vi "Get GPU Device Information.vi"(8 "error in":errorcluster, 9 "Reset Device?":bool, 10 "Test Device Execution?":bool, 11 "Device ID":T2) -> (0 "error out":errorcluster, 1 "CUDA Driver Version":string, 2 "CUDA Runtime API Version":string, 3 "Device Name":string, 4 "Supports Double Precision?":bool, 5 "Device Properties":T3[](array[typedef]), 7 "Available Devices":i32)   [LabVIEW 2020]
doc: "Investigates GPU devices installed in the system and optionally executes code on one of those devices."
uses:
  <vilib>/addons/lvgpu/lvcuda/CUDA Device (CUdevice).ctl
  <vilib>/addons/lvgpu/lvcuda/CUDA Device Properties (cudaDeviceProp).ctl
  <vilib>/addons/lvgpu/lvcuda.lvlib
  Get GPU Device Information.lvlib
panel:
  out "Status:":string
  in  "UI":T1(tab)
  out "Device Execution Profile":dbl[](graph)
  out "CUDA Build Version":string
  out "Error Help":string
  # "."
  # "The CUDA Runtime API version is the same as the CUDA Toolkit version. When multiple CUDA Toolkit versions are installed on the system, the inputs to Initialize Device or Initialize Library function determine which version is used. \n\nNOTE: This example uses the version selected when running Initialize Device with default inputs."
  # "The CUDA Driver version is determined by the NVIDIA display driver active in the OS."
  # "The CUDA Build version is the version of the CUDA Toolkit on which this toolkit's interface and settings are based."
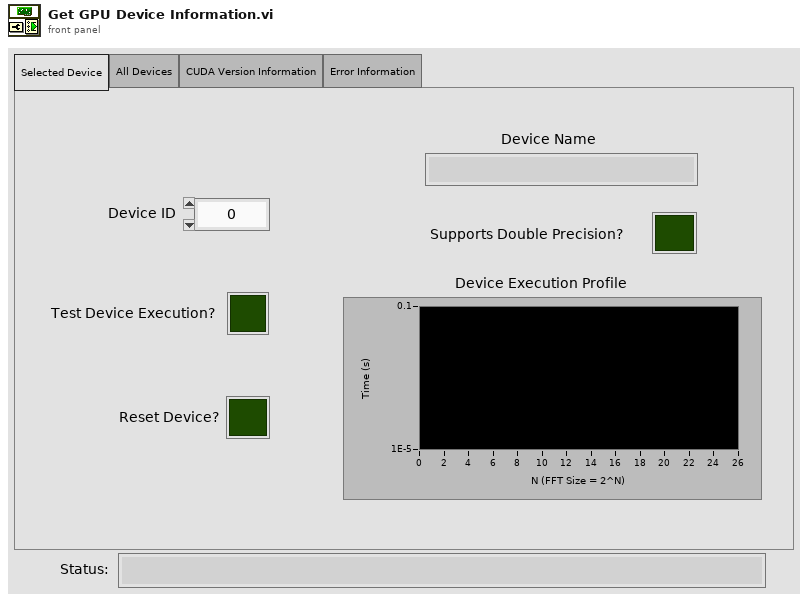
[diagram p1: front panel]
types:
  T1 = enum32{"Selected Device", "All Devices", "CUDA Version Information", "Error Information"}
  T2 = typedef "lvcuda.lvlib/CUDA Device (CUdevice).ctl" = i32
  T3 = typedef "lvcuda.lvlib/CUDA Device Properties (cudaDeviceProp).ctl" = cluster{"Name":string, "Total Global Memory (Bytes)":i64, "Shared Memory / Block (Bytes)":i32, "Registers / Block":i32, "Warp Size":i32, "Memory Pitch (Bytes)":i32, "Max Threads / Block":i32, "Max Threads Dim":i32[], "Max Grid Size":i32[], "Total Constant Memory":i32, "Major":i32, "Minor":i32, "Clock Rate (Hz)":i32, "Texture Alignment (Bytes)":i32}
  T4 = enum32{"Selected Device", "All Devices", "CUDA Version Information", "Error Information"}[]
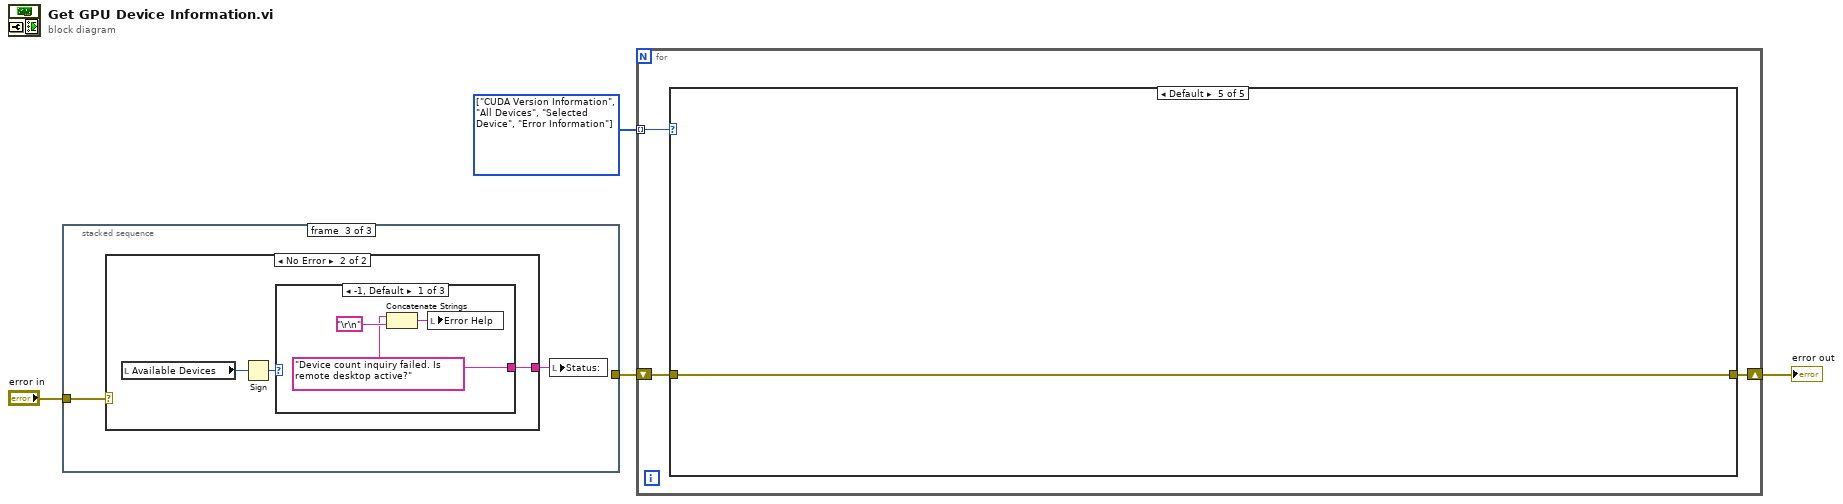
[diagram p0: block diagram]
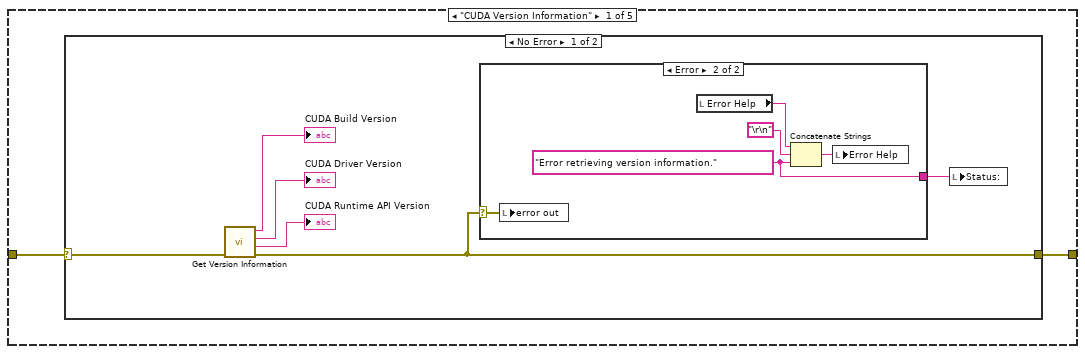
[diagram p2: hidden frame]
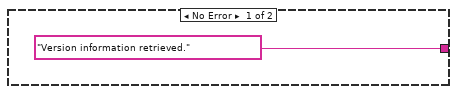
[diagram p3: hidden frame]
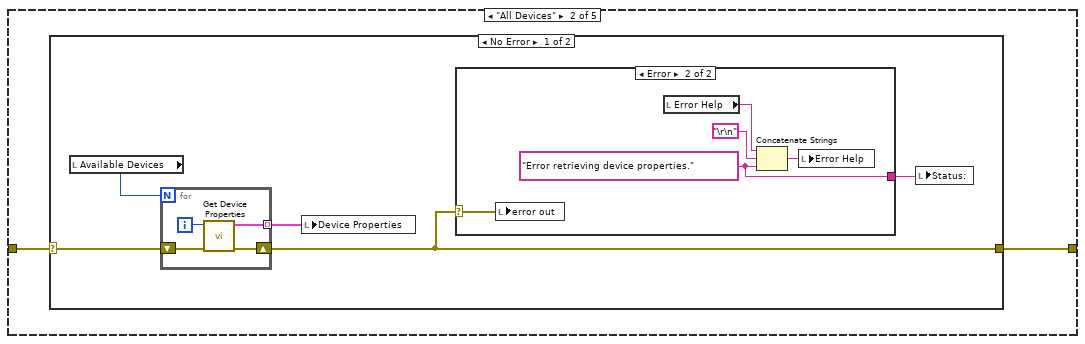
[diagram p5: hidden frame]
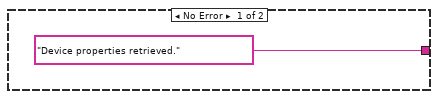
[diagram p6: hidden frame]
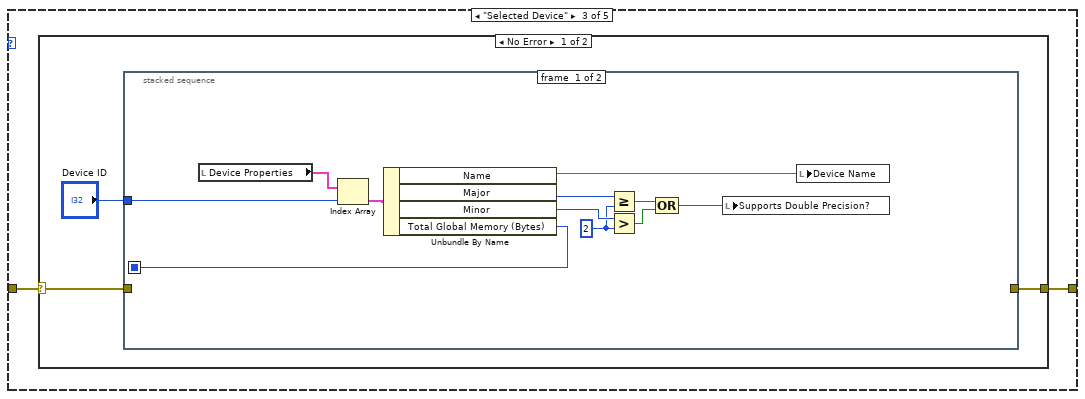
[diagram p8: hidden frame]
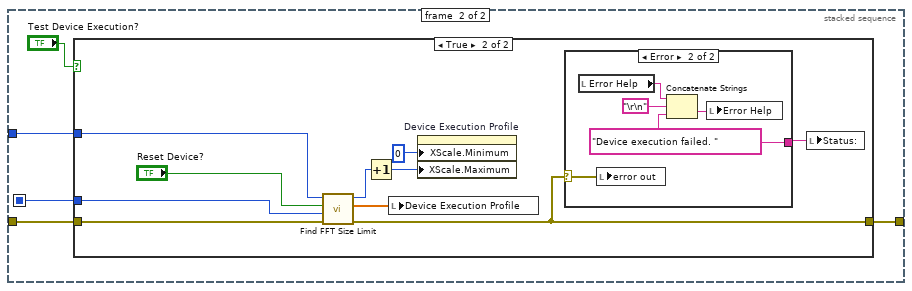
[diagram p9: hidden frame]
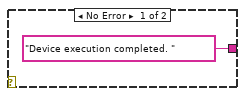
[diagram p11: hidden frame]
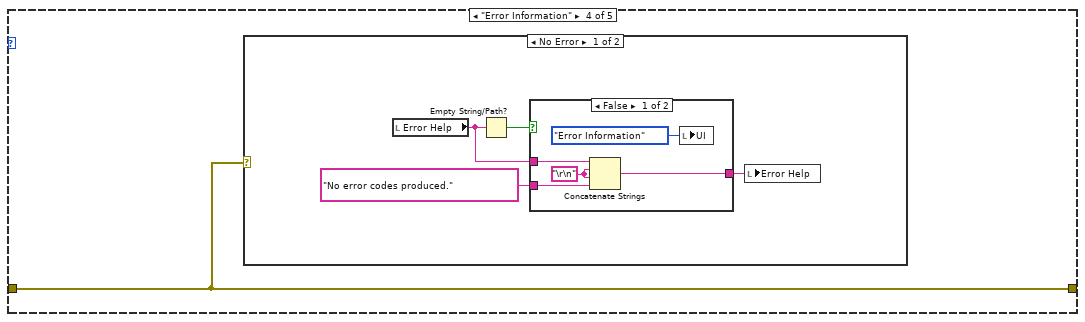
[diagram p13: hidden frame]
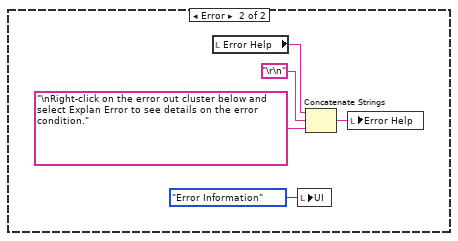
[diagram p15: hidden frame]
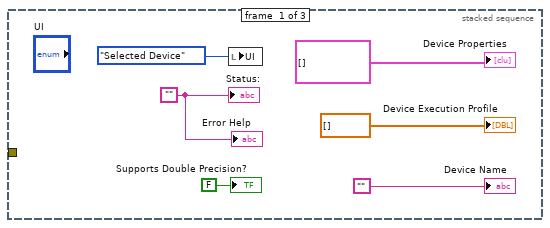
[diagram p16: hidden frame]
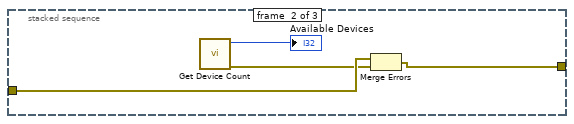
[diagram p17: hidden frame]
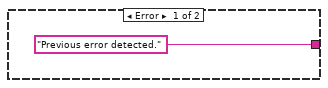
[diagram p18: hidden frame]
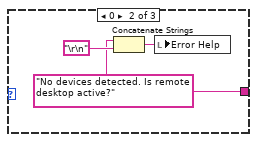
[diagram p19: hidden frame]
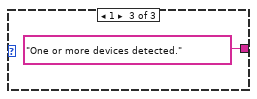
[diagram p20: hidden frame]
diagram:
  w1 = T4 [enum."CUDA Version Information", enum."All Devices", enum."Selected Device", enum."Error Information"] items=["Selected Device", "All Devices", "CUDA Version Information", "Error Information"]
  n1 = stacked-sequence {
    tunnel: [_ w13 _] -> w4
    tunnel: "error in" -> [_ w14 w16]
    frame #0 {
      w6 = ""
      n2 = local write "UI"(T1."Selected Device" ("UI")) -> ()
      "Status:" <- w6
      "Device Properties" <- T3[] [] ("Device Properties")
      "Device Execution Profile" <- dbl[] []
      "Supports Double Precision?" <- FALSE ("Supports Double Precision?")
      "Device Name" <- ""
      "Error Help" <- w6
    }
    frame #1 {
      n3 = call <vilib>:"Get Device Count.vi"() -> ("error out"=w12:errorcluster, "Number of CUDA Devices"=→"Available Devices":i32)  [unwired: 10 in]
      n4 = Merge Errors(w14, w12) -> (w13:errorcluster)
    }
    frame #2 {
      n5 = case shown="No Error" w16 {
        tunnel: ["Previous error detected." ("t") w19] -> w15
        frame Error {
        }
        frame No Error {
          n6 = local read "Available Devices"() -> (w18:i32)
          n7 = Sign(1:w18) -> (0:w20:i32)
          n8 = case shown="-1, Default" w20 {
            tunnel: [w21 w24 "One or more devices detected." ("t")] -> w19
            frame -1, Default {
              w21 = "Device count inquiry failed. Is remote desktop active?" ("t")
              n9 = Concatenate Strings(w21, "\r\n") -> (w23:string)
              n10 = local write "Error Help"(w23) -> ()
            }
            frame 0 {
              w24 = "No devices detected. Is remote desktop active?" ("t")
              n11 = Concatenate Strings(w24, "\r\n") -> (w26:string)
              n12 = local write "Error Help"(w26) -> ()
            }
            frame 1 {
            }
          }
        }
      }
      n13 = local write "Status:"(w15) -> ()
    }
  }
  n14 = for {
    tunnel: w1 -> [w28] mode=indexing
    shift-right: [w29] -> w3
    shift-left: w4 -> [w30]
    n15 = case shown="Default" w28 {
      tunnel: w30 -> [w31 w47 w65 w103 w119]
      tunnel: [w32 w46 w64 w103 w119] -> w29
      frame "CUDA Version Information" {
        n16 = case shown="No Error" w31 {
          selector: w31 -> [w38 w45]
          tunnel: [w37 w45] -> w32
          frame No Error {
            n17 = call <vilib>:"Get Version Information.vi"("error in"=w38) -> ("error out"=w37:errorcluster, "CUDA Runtime version"=→"CUDA Runtime API Version":string, "CUDA Driver version"=→"CUDA Driver Version":string, "CUDA Build version"=→"CUDA Build Version":string)  [unwired: 7 in]
            n18 = case shown="Error" w37 {
              selector: w37 -> [_ w44]
              tunnel: ["Version information retrieved." ("Status") w40] -> w33
              frame No Error {
              }
              frame Error {
                w40 = "Error retrieving version information." ("Status")
                n19 = local write "error out"(w44) -> ()
                n20 = local read "Error Help"() -> (w42:string)
                n21 = Concatenate Strings(w42, "\r\n", w40) -> (w43:string)
                n22 = local write "Error Help"(w43) -> ()
              }
            }
            n23 = local write "Status:"(w33) -> ()
          }
          frame Error {
          }
        }
      }
      frame "All Devices" {
        n24 = case shown="No Error" w47 {
          selector: w47 -> [w52 w63]
          tunnel: [w49 w63] -> w46
          frame No Error {
            n25 = local read "Available Devices"() -> (w51:i32)
            n26 = for {
              N: w51 -> [_]
              shift-right: [w61] -> w49
              shift-left: w52 -> [w62]
              tunnel: [w59] -> w50 mode=indexing
              i -> [w60]
              n27 = call <vilib>:"Get Device Properties.vi"("error in"=w62, "device"=w60) -> ("error out"=w61:errorcluster, "CUDA Device Properties"=w59:T3)  [unwired: 8 in]
            }
            n28 = local write "Device Properties"(w50) -> ()
            n29 = case shown="Error" w49 {
              selector: w49 -> [_ w58]
              tunnel: ["Device properties retrieved." w54] -> w48
              frame No Error {
              }
              frame Error {
                w54 = "Error retrieving device properties."
                n30 = local write "error out"(w58) -> ()
                n31 = local read "Error Help"() -> (w56:string)
                n32 = Concatenate Strings(w56, "\r\n", w54) -> (w57:string)
                n33 = local write "Error Help"(w57) -> ()
              }
            }
            n34 = local write "Status:"(w48) -> ()
          }
          frame Error {
          }
        }
      }
      frame "Selected Device" {
        n35 = case shown="No Error" w65 {
          selector: w65 -> [w68 w102]
          tunnel: [w67 w102] -> w64
          frame No Error {
            n36 = stacked-sequence {
              seq-local: [w69 _] -> [_ w80]
              tunnel: w68 -> [_ w83]
              tunnel: [_ w82] -> w67
              tunnel: "Device ID" -> [w72 w81]
              frame #0 {
                w76 = 2 ("y")
                n37 = local read "Device Properties"() -> (w79:T3[])
                n38 = Index Array(array=w79, index=w72) -> (element=w73:T3)
                n39 = Unbundle By Name(w73) -> ("Name"=w70:string, "Major"=w78:i32, "Minor"=w77:i32, "Total Global Memory (Bytes)"=w69:i64)
                n40 = Greater Or Equal?(x=w78, y=w76) -> (x >= y?=w75:bool)
                n41 = Greater?(x=w77, y=w76) -> (0:w74:bool)
                n42 = Compound Arithmetic op=OR(w75, w74) -> (w71:bool)
                n43 = local write "Supports Double Precision?"(w71) -> ()
                n44 = local write "Device Name"(w70) -> ()
              }
              frame #1 {
                n45 = case shown="True" "Test Device Execution?" {
                  tunnel: w83 -> [w85 w95]
                  tunnel: [w85 w91] -> w82
                  tunnel: w81 -> [_ w88]
                  tunnel: w80 -> [_ w86]
                  frame False {
                  }
                  frame True {
                    n46 = call "Find FFT Size Limit.vi"("error in"=w95, "Total Global Memory (Bytes)"=w86, "Reset Device?"="Reset Device?", "Device ID"=w88) -> ("error out"=w91:errorcluster, "FFT Execution Times (s)"=w90:dbl[], "N"=w89:i32)  [unwired: 5 in]
                    n47 = Increment(x=w89) -> (x+1=w87:i32)
                    n48 = local write "Device Execution Profile"(w90) -> ()
                    n49 = property on="Device Execution Profile" class="WFGraph (strict)"("XScale.Minimum"=0 ("N"), "XScale.Maximum"=w87) -> ()  [unwired: 2 in, 2 out]
                    n50 = case shown="Error" w91 {
                      selector: w91 -> [_ w101]
                      tunnel: ["Device execution completed. " ("Name") w97] -> w93
                      frame No Error {
                      }
                      frame Error {
                        w97 = "Device execution failed. " ("Name")
                        n51 = local read "Error Help"() -> (w99:string)
                        n52 = local write "error out"(w101) -> ()
                        n53 = Concatenate Strings(w99, "\r\n", w97) -> (w100:string)
                        n54 = local write "Error Help"(w100) -> ()
                      }
                    }
                    n55 = local write "Status:"(w93) -> ()
                  }
                }
              }
            }
          }
          frame Error {
          }
        }
      }
      frame "Error Information" {
        n56 = case shown="No Error" w103 {
          frame No Error {
            n57 = local read "Error Help"() -> (w106:string)
            n58 = Empty String/Path?(string/path=w106) -> (empty?=w105:bool)
            n59 = case shown="False" w105 {
              tunnel: w106 -> [w112 _]
              tunnel: [w111 w113] -> w107
              tunnel: "No error codes produced." ("Error String") -> [w109 w113]
              frame False {
                w110 = "\r\n"
                n60 = Concatenate Strings(w112, w110, w110, w109) -> (w111:string)
                n61 = local write "UI"(T1."Error Information" ("UI")) -> ()
              }
              frame True {
              }
            }
            n62 = local write "Error Help"(w107) -> ()
          }
          frame Error {
            n63 = local read "Error Help"() -> (w117:string)
            n64 = local write "UI"(T1."Error Information" ("UI")) -> ()
            n65 = Concatenate Strings(w117, "\r\n", "\nRight-click on the error out cluster below and select Explan Error to see details on the error condition." ("Error Help")) -> (w115:string)
            n66 = local write "Error Help"(w115) -> ()
          }
        }
      }
      frame Default {
      }
    }
  }
  "error out" <- w3
